vi "saveDataNodeBegin.vi"(8 "error in (no error)":errorcluster, 9 "indent":i32, 10 "XML Refnum in":refnum<file>, 11 "DMA_Write in":refnum<class "DMA_Write.lvclass">) -> (0 "error out":errorcluster, 2 "XML Refnum out":refnum<file>, 3 "DMA_Write out":refnum<class "DMA_Write.lvclass">)   [LabVIEW 2013, in "DMA_Write.lvclass"]
doc: "Begins the process of saving a xceData Node to an XML formatted file."
uses:
  DMA_Write.lvclass
  xCE/xceNode/xceNode.lvclass
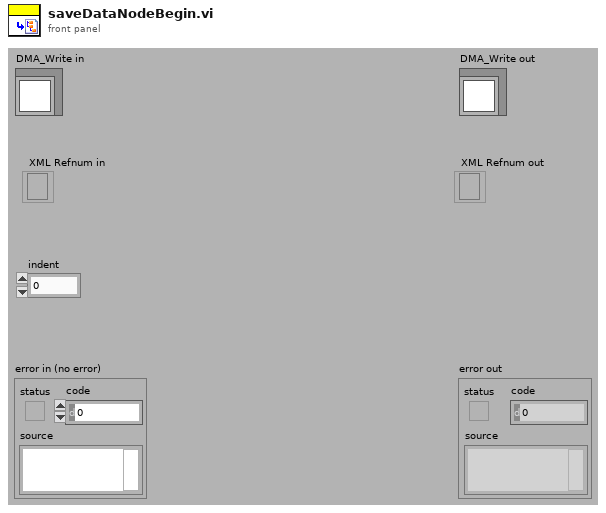
[diagram p1: front panel]
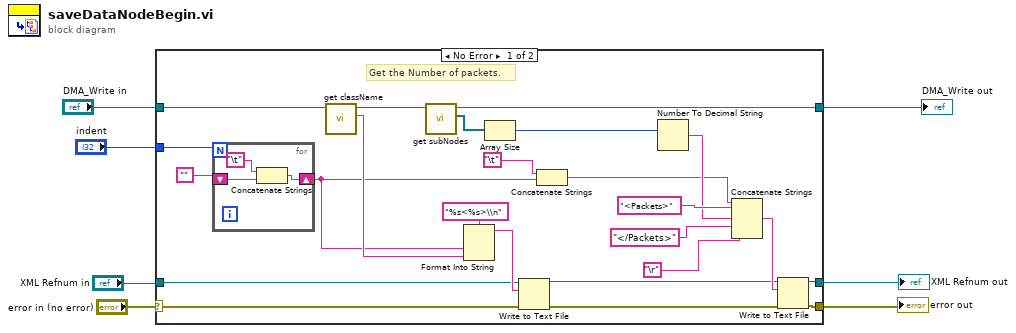
[diagram p0: block diagram]
diagram:
  n1 = case shown="No Error" "error in (no error)" {
    selector: "error in (no error)" -> [w16 w37]
    tunnel: "XML Refnum in" -> [w17 w36]
    tunnel: [w23 w37] -> w4
    tunnel: [w24 w36] -> w5
    tunnel: "DMA_Write in" -> [w21 w35]
    tunnel: [w9 w35] -> w6
    tunnel: "indent" -> [w30 _]
    frame No Error {
      # "Get the Number of packets."
      n2 = for {
        N: w30 -> [_]
        shift-right: [w34] -> w19
        shift-left: "" -> [w33]
        n3 = Concatenate Strings("\t", w33) -> (w34:string)
      }
      n4 = call "get className.vi"("xceNode in"=w21) -> ("Class name"=w20:string, "xceNode out"=w10:refnum<class "DMA_Write.lvclass">)  [unwired: 8 in, 1 out]
      n5 = call "get subNodes.vi"("xceNode in"=w10) -> ("subNodes[]*"=w11:refnum<data-value>[], "xceNode out"=w9:refnum<class "DMA_Write.lvclass">)  [unwired: 8 in, 1 out]
      n6 = Format Into String(format string="%s<%s>\\n", w19, w20) -> (resulting string=w18:string)  [unwired: 2 in, 1 out]
      n7 = Array Size(array=w11) -> (size(s)=w8:i32)
      n8 = Write to Text File(file (use dialog)=w17, text=w18, error in=w16) -> (refnum out=w15:refnum<file>, error out=w14:errorcluster)  [unwired: 1 in, 1 out]
      n9 = Concatenate Strings("\t", w19) -> (w12:string)
      n10 = Number To Decimal String(number=w8) -> (decimal integer string=w26:string)  [unwired: 1 in]
      n11 = Concatenate Strings(w12, "<Packets>" ("string"), w26, "</Packets>" ("string"), "\r") -> (w25:string)
      n12 = Write to Text File(file (use dialog)=w15, text=w25, error in=w14) -> (refnum out=w24:refnum<file>, error out=w23:errorcluster)  [unwired: 1 in, 1 out]
    }
    frame Error {
    }
  }
  "error out" <- w4
  "DMA_Write out" <- w6
  "XML Refnum out" <- w5
